vi "Child Handshake CC.vi"(8 "error in (no error)":errorcluster, 10 "Child Core Data":T1, 11 "Camera Controller in":refnum<class "Camera Controller.lvclass">) -> (0 "error out":errorcluster, 3 "Camera Controller out":refnum<class "Camera Controller.lvclass">)   [LabVIEW 2019, in "Camera Controller.lvlib" / "Camera Controller.lvclass"]
uses:
  Camera Controller.lvclass
  <vilib>/ActorFramework/Message Enqueuer/Message Enqueuer.lvclass
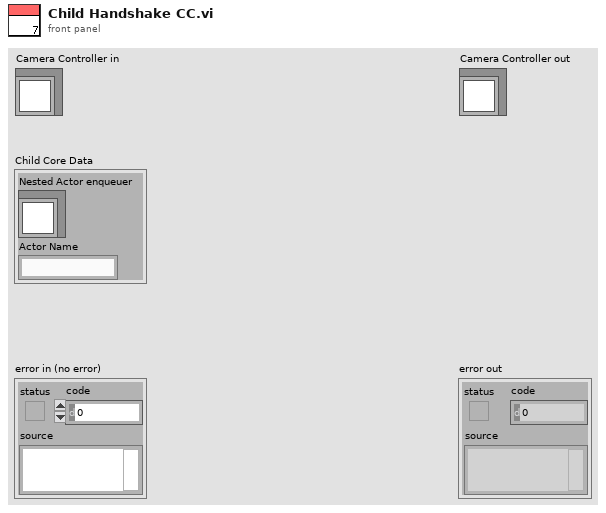
[diagram p1: front panel]
types:
  T1 = cluster{"Nested Actor enqueuer":refnum<class "Message Enqueuer.lvclass">, "Actor Name":string}
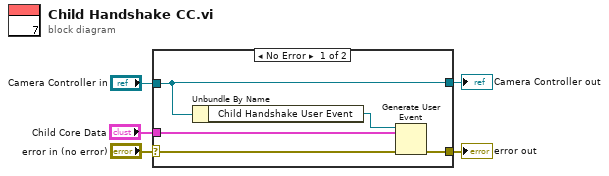
[diagram p0: block diagram]
diagram:
  n1 = case shown="No Error" "error in (no error)" {
    selector: "error in (no error)" -> [w10 w12]
    tunnel: [w9 w12] -> w4
    tunnel: [w8 w11] -> w2
    tunnel: "Camera Controller in" -> [w8 w11]
    tunnel: "Child Core Data" -> [w6 _]
    frame No Error {
      n2 = Unbundle By Name(w8) -> ("Child Handshake User Event"=w7:refnum<user-event>)
      n3 = Generate User Event(user event=w7, event data cluster=w6, error in=w10) -> (error out=w9:errorcluster)  [unwired: 1 in, 1 out]
    }
    frame Error {
    }
  }
  "error out" <- w4
  "Camera Controller out" <- w2
